vi "Performance Test.vi"() -> ()   [LabVIEW 2021]
uses:
  CIFChannels/Typedef/Direction.ctl
  CIF_NIChn_Fifo_Power.lvclass
  D:/dev/CIF-LVCore/src/Channels/CIFChannels/CIFChannels.lvclass
  D:/dev/CIF-LVCore/src/Channels/CIF_NIChn/NIChn/CIF_NIChn.lvclass
  ChannelCommon/typedef/FIFO Config.ctl
  <vilib>/Platform/TimedLoop/XDataNode/timing_clust.ctl
  <vilib>/Platform/TimedLoop/XDataNode/nitl_modes.ctl
  <vilib>/Platform/TimedLoop/XDataNode/wakeup.ctl
  ChannelCommon/typedef/Datatype Waveform.ctl
  CIF_NIChn_Fifo_Power.lvclass/CIF_NIChn_Fifo_Power.ctl
  ChannelCommon/CIFFIFO/CIFfifo.lvclass/CIFfifo.ctl
  NIChn/CIF_NIChn.lvclass/CIF_NIChn.ctl
  CIFChannels/CIFChannels.lvclass/CIFChannels.ctl
  CIFCore/Common/Utilities/Add Error.vi
  SubVIs/Add Error.vi
  <vilib>/CIFChannels/Top Level/Write Variable Length U8 Array.vi
  NIChn/Accessors/Read CIF Channel.vi
  NIChn/Accessors/Write CIF Channel.vi
  SubVIs/Flatten.vi
  ChannelCommon/CIFFIFO/Accessors/Read Length.vi
  NIChn/SubVIs/Check Disconnect.vi
  <vilib>/CIFChannels/Top Level/Read Variable Length U8 Array.vi
  SubVIs/Unflatten.vi
  CIFChannels/Accessors/Read Channel State.vi
  CIFChannels/Accessors/Read Direction.vi
  CIFCore/Common/Utilities/Append Error Location.vi
  <vilib>/CIFChannels/SubVIs/Get dll Path.vi
  ChannelCommon/CIFFIFO/Utilities/Update Header.vi
  ChannelCommon/CIFFIFO/Flatten/Waveform Flatten.vi
  ChannelCommon/CIFFIFO/Accessors/Write T0.vi
  ChannelCommon/CIFFIFO/Accessors/Write T_Out.vi
  CIFChannels/Accessors/Write Channel State.vi
  CIFChannels/Accessors/Read Disconnect Behavior.vi
  <vilib>/CIFChannels/Top Level/Read Variable Length U8 Array.vi/81056090-23cf-424a-a716-29db01c8ef1b.vi
  <vilib>/CIFChannels/Top Level/Read Variable Length U8 Array.vi/6610cd62-0a6d-4591-8fd4-6453482a4bc1.vi
  <vilib>/CIFChannels/Top Level/Read Variable Length U8 Array.vi/93d598b0-524b-4f76-9570-a74a86ef2c6f.vi
  ChannelCommon/CIFFIFO/Accessors/Write Timeout.vi
  ChannelCommon/CIFFIFO/Flatten/Waveform Unflatten.vi
  ChannelCommon/CIFFIFO/Accessors/Read Header.vi
  ChannelCommon/CIFFIFO/Accessors/Write Header.vi
  ChannelCommon/Utilities/Flatten Header.vi
  ChannelCommon/CIFFIFO/Flatten/Waveform Flatten.vi/6fdbece9-bad6-4a8e-9bf7-fe1528478dd6.vi
  ChannelCommon/CIFFIFO/Flatten/Waveform Flatten.vi/d5e54e4f-7f1a-40ef-960c-6b2cd585230c.vi
  ChannelCommon/CIFFIFO/Flatten/Waveform Flatten.vi/a071385d-aa0c-48d2-a5ce-3b08816305e6.vi
  ChannelCommon/CIFFIFO/Accessors/Write Payload Length.vi
  <vilib>/CIFChannels/Top Level/Read Variable Length U8 Array.vi/81056090-23cf-424a-a716-29db01c8ef1b.vi/4bc1c15b-36ab-481f-b8dd-c64075ce723a.vi
  <vilib>/CIFChannels/Top Level/Read Variable Length U8 Array.vi/81056090-23cf-424a-a716-29db01c8ef1b.vi/d83cb72b-7713-41fc-a3d1-682de79cf574.vi
  <vilib>/CIFChannels/Top Level/Read Variable Length U8 Array.vi/6610cd62-0a6d-4591-8fd4-6453482a4bc1.vi/c28b0ead-42ad-4072-80a2-aca7f2bd7ce3.vi
  <vilib>/CIFChannels/Top Level/Read Variable Length U8 Array.vi/93d598b0-524b-4f76-9570-a74a86ef2c6f.vi/4bc1c15b-36ab-481f-b8dd-c64075ce723a.vi
  <vilib>/CIFChannels/Top Level/Read Variable Length U8 Array.vi/93d598b0-524b-4f76-9570-a74a86ef2c6f.vi/d83cb72b-7713-41fc-a3d1-682de79cf574.vi
  ChannelCommon/Utilities/Unflatten Header.vi
  ChannelCommon/CIFFIFO/Flatten/Waveform Flatten.vi/6fdbece9-bad6-4a8e-9bf7-fe1528478dd6.vi/c28b0ead-42ad-4072-80a2-aca7f2bd7ce3.vi
  ChannelCommon/CIFFIFO/Flatten/Waveform Flatten.vi/d5e54e4f-7f1a-40ef-960c-6b2cd585230c.vi/c28b0ead-42ad-4072-80a2-aca7f2bd7ce3.vi
  ChannelCommon/CIFFIFO/Flatten/Waveform Flatten.vi/a071385d-aa0c-48d2-a5ce-3b08816305e6.vi/c28b0ead-42ad-4072-80a2-aca7f2bd7ce3.vi
  NIChn/CIF_NIChn.lvclass
  ChannelCommon/Utilities/Update Time.vi
  <vilib>/Platform/TimedLoop/XDataNode/XDataNode.xnode
  <vilib>/Platform/TimedLoop/XDataNode/XDNodeRunTimeDep.lvlib
  CIFChannels/CIFChannels.lvclass
  ChannelCommon/ChannelCommon.lvlib
panel:
  out "avg big channel":dbl
  out "max big channel":dbl
  out "timed out? 4":bool
  out "avg TO":dbl
  out "max TO":dbl
  out "timed out? 3":bool
  out "avg Direct":dbl
  out "max Direct":dbl
  out "timed out? 2":bool
  out "timed out?":bool
  out "avg channel":dbl
  out "max channel":dbl
  out "pass":bool
  out "error out":errorcluster
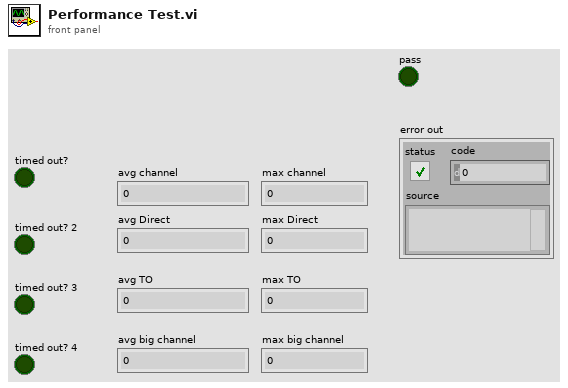
[diagram p1: front panel]
types:
  T1 = typedef "ChannelCommon.lvlib/FIFO Config.ctl" = cluster{"Depth":u64, "Flags":u64, "ClockID":u8}
  T2 = typedef "CIFChannels.lvclass/Direction.ctl" = enum16{"Publisher", "Subscriber"}
  T3 = typedef "ChannelCommon.lvlib/Datatype Waveform.ctl" = cluster{"measurement":dbl[], "dT":dbl, "Timestamp":u64}
  T4 = typedef "XDNodeRunTimeDep.lvlib/timing_clust.ctl" = cluster{"Expected End [f-1]":u64, "Actual End [f-1]":u64, "Finished Late? [f-1]":bool, "Expected End [i-1]":u64, "Actual End [i-1]":u64, "Finished Late? [i-1]":bool, "Expected Start [i]":u64, "Actual Start [i]":u64, "Expected Start [f]":u64, "Actual Start [f]":u64, "Source Name":string, "Structure Name":string, "Period":i64, "Deadline":i64, "Offset":i64, "Start":i64, "Priority":i32, "Timeout":i32, "Mode":T5, "Wakeup Reason":T6, "Error":errorcluster, "Source Type":string, "Secondary Source Type":string, "Global End Time":u64, "Global Start Time":u64, "Frame Duration":u64, "Iteration Duration":u64, "Assigned CPU":i32, "I/O Scan Engine Mode":u32}
  T5 = typedef "XDNodeRunTimeDep.lvlib/nitl_modes.ctl" = enum32{"No Change", "Process missed periods, maintain original phase", "Discard missed periods, maintain original phase", "Process missed periods, ignore original phase", "Discard missed periods, ignore original phase"}
  T6 = typedef "XDNodeRunTimeDep.lvlib/wakeup.ctl" = enum32{"Normal", "Aborted", "Asynchronous wakeup", "Timing source error", "Timed loop error", "Timeout"}
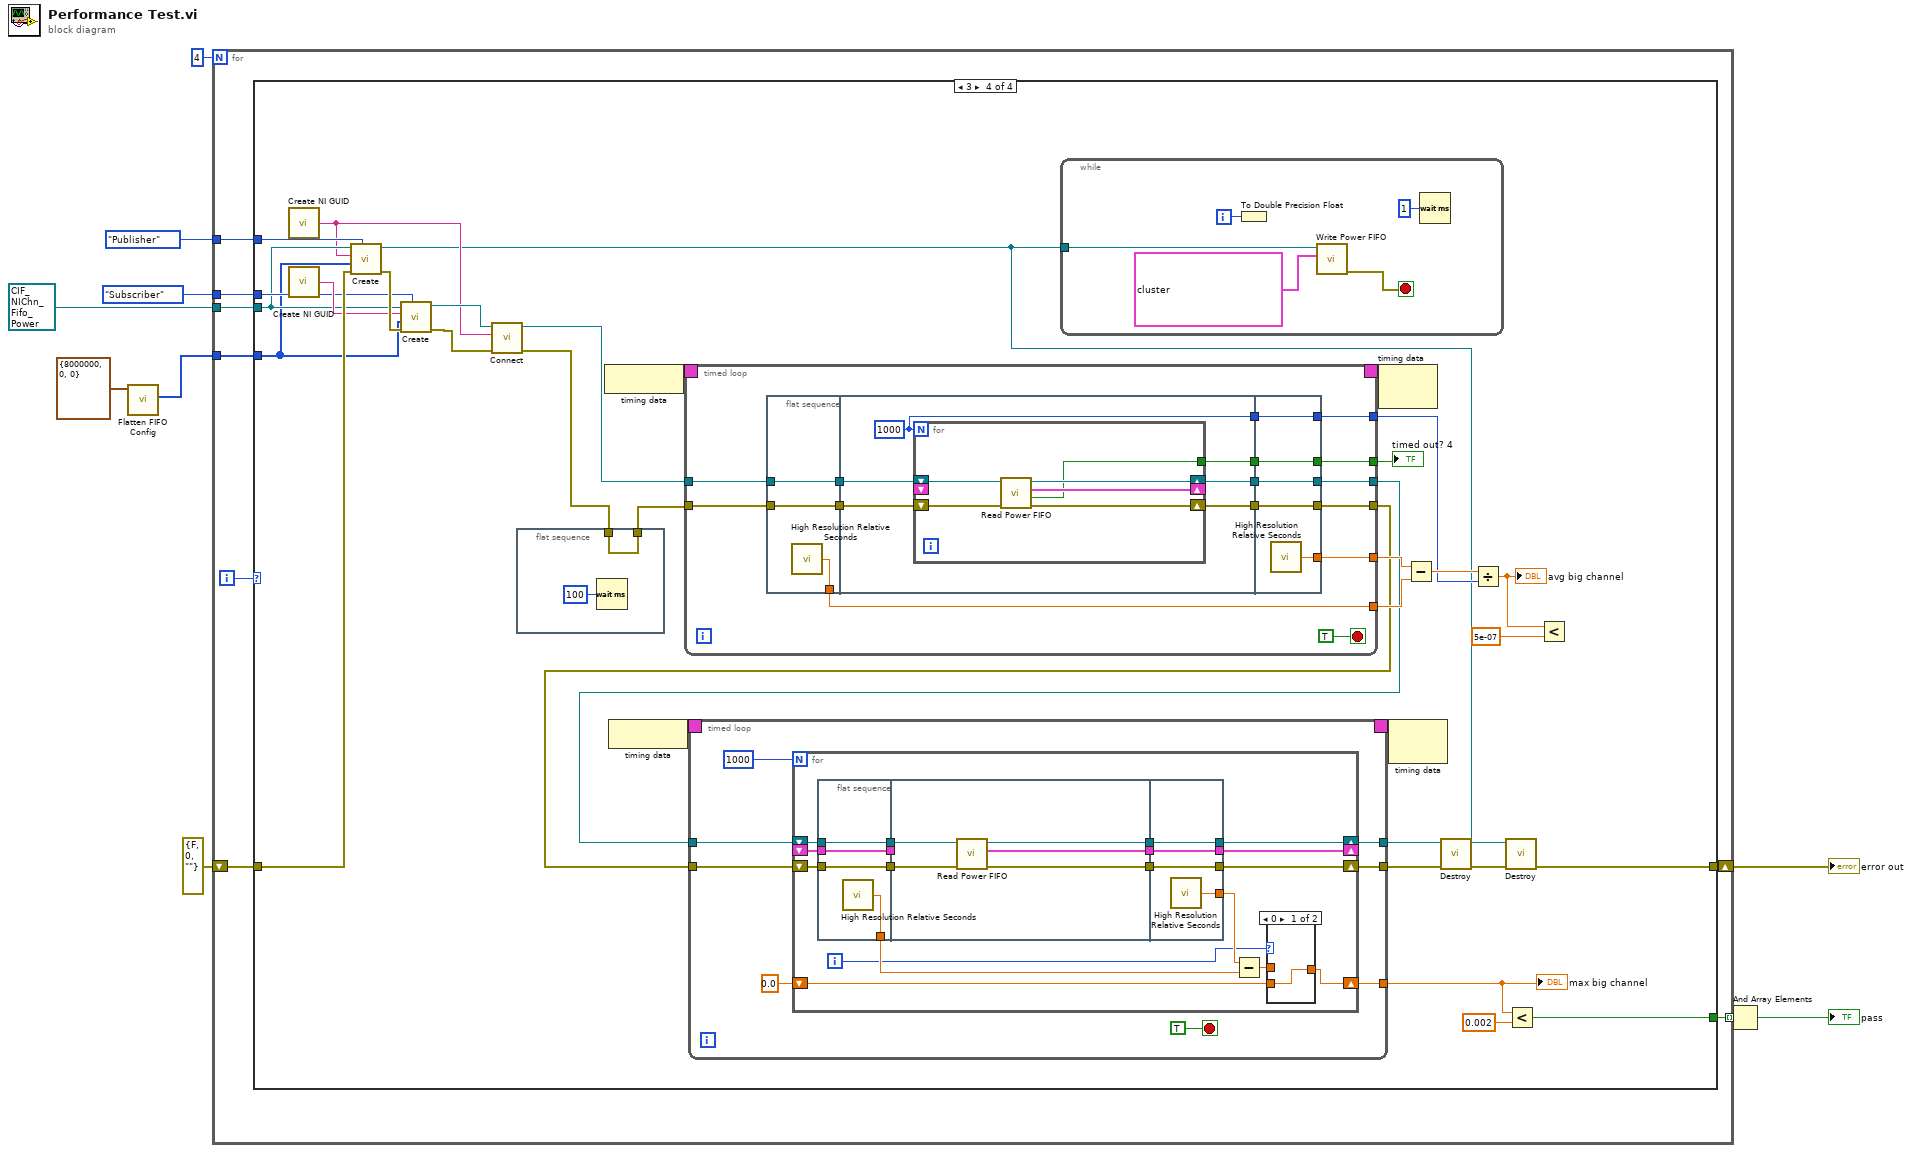
[diagram p0: block diagram]
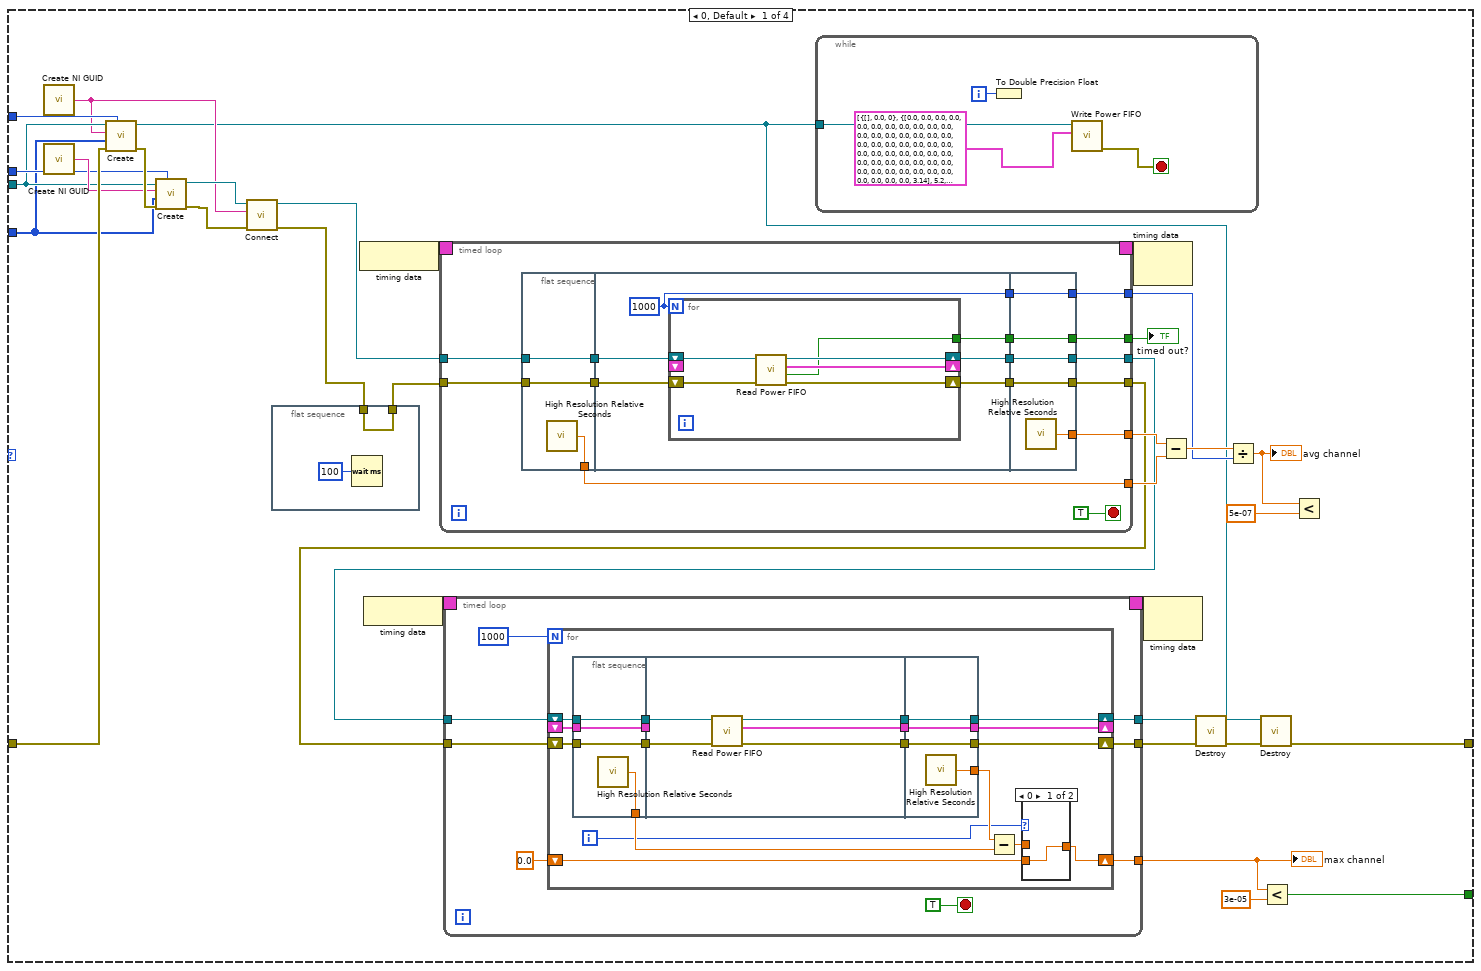
[diagram p2: hidden frame]
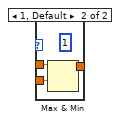
[diagram p3: hidden frame]
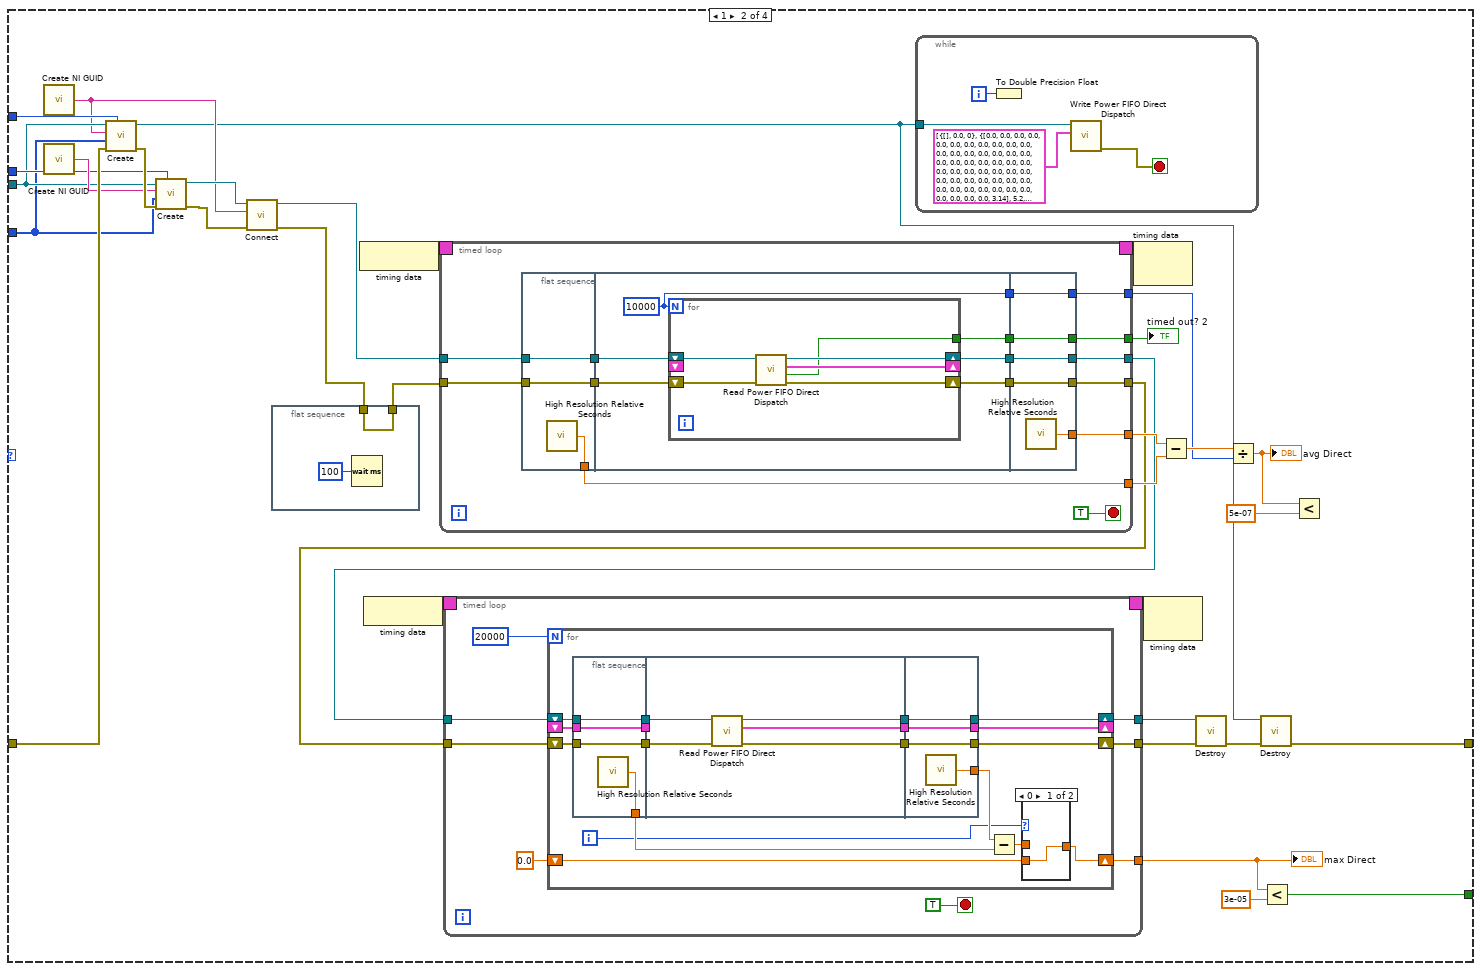
[diagram p4: hidden frame]
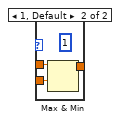
[diagram p5: hidden frame]
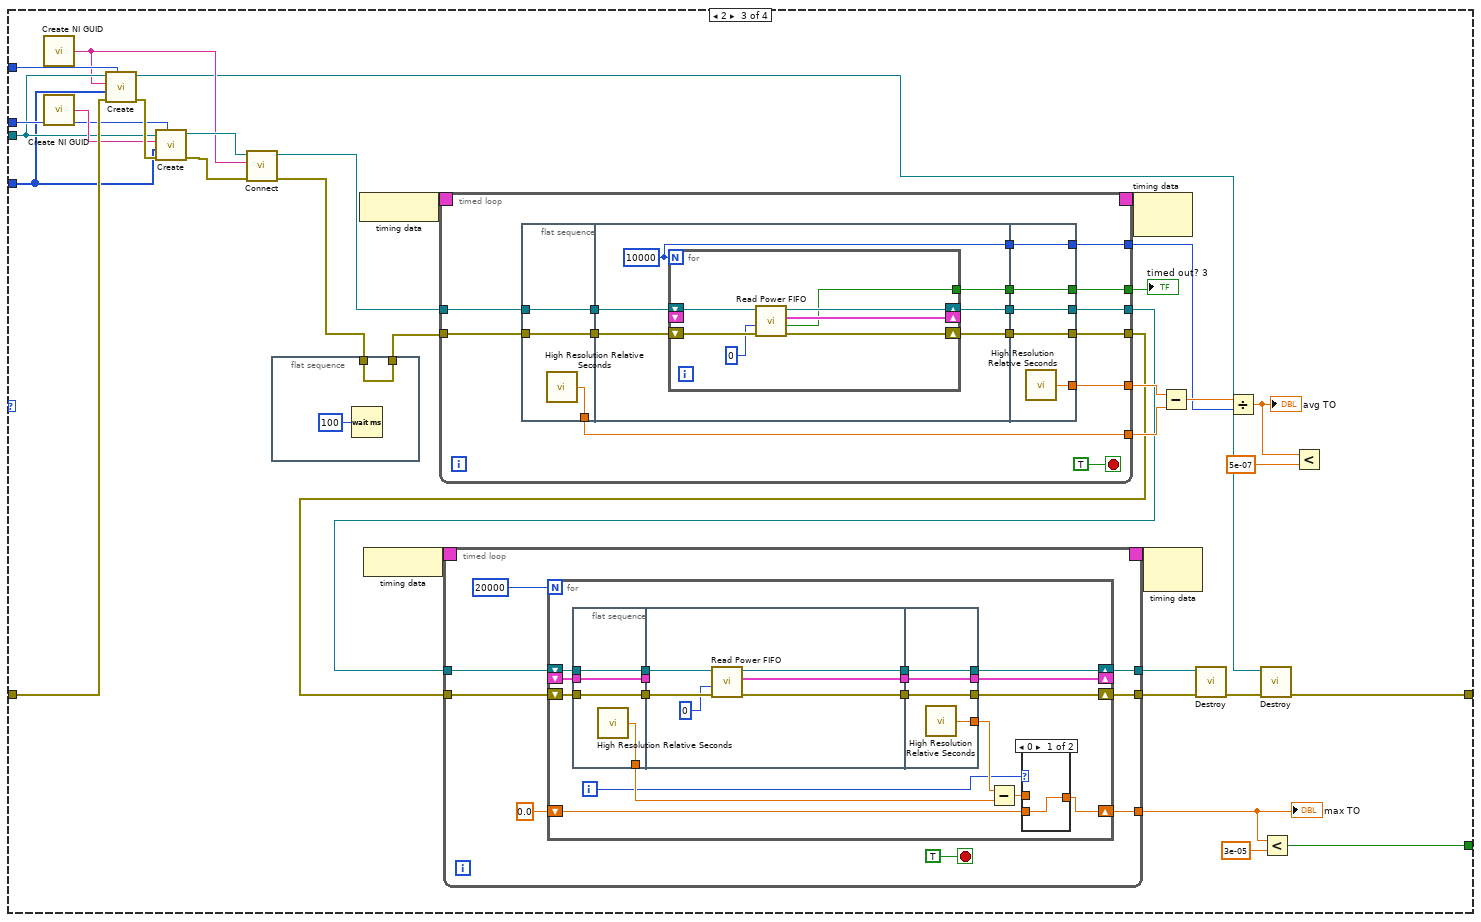
[diagram p6: hidden frame]
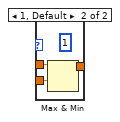
[diagram p7: hidden frame]
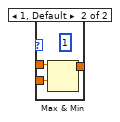
[diagram p8: hidden frame]
diagram:
  n1 = call "Flatten FIFO Config.vi"("FIFO Config in"=T1 {"Depth"=8000000, "Flags"=0, "ClockID"=0}) -> ("Flattened Data out"=w2:u8[])  [unwired: 8 in, 2 out]
  n2 = for {
    N: 4 -> [_]
    tunnel: [w18] -> w8 mode=indexing
    shift-right: [w17] -> w10
    shift-left: errorcluster {"status"=FALSE, "code"=0, "source"=""} ("error out") -> [w15]
    tunnel: Direction."Publisher" ("Direction") -> [w14]
    tunnel: Direction."Subscriber" ("Direction") -> [w13]
    tunnel: refnum<class "CIF_NIChn_Fifo_Power.lvclass"> refnum ("CIF_NIChn_Fifo_Power.lvclass") -> [w12]
    tunnel: w2 -> [w11]
    i -> [w16]
    n3 = case shown="3" w16 {
      tunnel: [w38 w164 w290 w414] -> w18
      tunnel: [w22 w148 w274 w398] -> w17
      tunnel: w15 -> [w36 w162 w288 w412]
      tunnel: w14 -> [w34 w160 w286 w410]
      tunnel: w13 -> [w33 w159 w285 w409]
      tunnel: w12 -> [w32 w158 w284 w408]
      tunnel: w11 -> [w28 w154 w280 w404]
      frame 0, Default {
        n4 = call <vilib>:"Create NI GUID.vi"() -> ("NI GUID"=w30:string)
        n5 = call <vilib>:"Create NI GUID.vi"() -> ("NI GUID"=w35:string)
        n6 = call-dynamic "Create.vi"("Direction"=w34, "error in (no error)"=w36, "Custom Config Data"=w28, "Name"=w30, "CIFTag in"=w32) -> ("error out"=w37:errorcluster, "CIFTag out"=w23:refnum<class "CIF_NIChn_Fifo_Power.lvclass">)  [unwired: 5 in]
        n7 = call-dynamic "Create.vi"("Direction"=w33, "error in (no error)"=w37, "Custom Config Data"=w28, "Name"=w35, "CIFTag in"=w32) -> ("error out"=w29:errorcluster, "CIFTag out"=w31:refnum<class "CIF_NIChn_Fifo_Power.lvclass">)  [unwired: 5 in]
        n8 = call-dynamic "Connect.vi"("error in (no error)"=w29, "Connection Name"=w30, "CIFTag in"=w31) -> ("error out"=w21:errorcluster, "CIFTag out"=w27:refnum<class "CIF_NIChn_Fifo_Power.lvclass">)  [unwired: 7 in]
        n9 = flat-sequence {
          tunnel: w21 -> [w54]
          tunnel: [w54] -> w20
          frame #0 {
            n10 = Wait (ms)(milliseconds to wait=u32 100) -> ()  [unwired: 1 out]
          }
        }
        n11 = node-c288() -> (w52:T4)
        n12 = node-c288() -> (w50:T4)
        n13 = timed-loop {
          timing: w52 -> [_]
          timing-out: [_] -> w51
          tunnel: w27 -> [w120]
          tunnel: w20 -> [w119]
          tunnel: [w115] -> w44
          tunnel: [w113] -> w43
          tunnel: [w111] -> w48
          tunnel: [w110] -> w47
          tunnel: [w109] -> w45
          tunnel: [w107] -> w19
          stop <- TRUE stop-if-true
          n14 = flat-sequence {
            tunnel: w119 -> [w122]
            tunnel: w120 -> [w123]
            tunnel: [w123] -> w117
            tunnel: [w122] -> w116
            tunnel: [w121] -> w110
            tunnel: w117 -> [w129]
            tunnel: w116 -> [w128]
            tunnel: [w127] -> w114
            tunnel: [w126] -> w112
            tunnel: [w125] -> w108
            tunnel: [w124] -> w106
            tunnel: [w140] -> w115
            tunnel: w114 -> [w140]
            tunnel: [w139] -> w113
            tunnel: w112 -> [w139]
            tunnel: [w138] -> w111
            tunnel: [w137] -> w109
            tunnel: w108 -> [w137]
            tunnel: [w136] -> w107
            tunnel: w106 -> [w136]
            frame #0 {
              n15 = call <vilib>:"High Resolution Relative Seconds.vi"() -> ("relative seconds"=w121:dbl)
            }
            frame #1 {
              w125 = 1000
              n16 = for {
                N: w125 -> [_]
                shift-right: [w134] -> w127
                shift-left: w129 -> [w135]
                shift-right: [w132] -> w126
                shift-left: w128 -> [w133]
                shift-right: [w131] -> _
                shift-left: _ -> [_]
                tunnel: [w130] -> w124
                n17 = call-dynamic "Read Power FIFO.vi"("error in (no error)"=w133, "CIFTag in"=w135) -> ("error out"=w132:errorcluster, "timed out?"=w130:bool, "Data out"=w131:T3[], "CIFTag out"=w134:refnum<class "CIF_NIChn_Fifo_Power.lvclass">)  [unwired: 5 in, 1 out]
              }
            }
            frame #2 {
              n18 = call <vilib>:"High Resolution Relative Seconds.vi"() -> ("relative seconds"=w138:dbl)
            }
          }
        }
        "timed out?" <- w19
        n19 = timed-loop {
          timing: w50 -> [_]
          timing-out: [_] -> w49
          tunnel: w44 -> [w66]
          tunnel: w43 -> [w65]
          tunnel: [w63] -> w26
          tunnel: [w62] -> w25
          tunnel: [w59] -> w40
          stop <- TRUE stop-if-true
          n20 = for {
            N: 1000 -> [_]
            shift-right: [w78] -> w63
            shift-left: w66 -> [w80]
            shift-right: [w77] -> w62
            shift-left: w65 -> [w79]
            shift-right: [w71] -> w59
            shift-left: 0.0 -> [w72]
            shift-right: [w70] -> _
            shift-left: _ -> [w76]
            i -> [w68]
            n21 = flat-sequence {
              tunnel: w79 -> [w91]
              tunnel: w80 -> [w92]
              tunnel: [w92] -> w84
              tunnel: [w91] -> w83
              tunnel: [w90] -> w74
              tunnel: w76 -> [w89]
              tunnel: [w89] -> w82
              tunnel: w84 -> [w97]
              tunnel: w83 -> [w95]
              tunnel: [w96] -> w81
              tunnel: w82 -> [_]
              tunnel: [w93] -> w69
              tunnel: [w94] -> w67
              tunnel: [w101] -> w78
              tunnel: w81 -> [w101]
              tunnel: [w100] -> w77
              tunnel: [w99] -> w75
              tunnel: [w98] -> w70
              tunnel: w69 -> [w98]
              tunnel: w67 -> [w100]
              frame #0 {
                n22 = call <vilib>:"High Resolution Relative Seconds.vi"() -> ("relative seconds"=w90:dbl)
              }
              frame #1 {
                n23 = call-dynamic "Read Power FIFO.vi"("error in (no error)"=w95, "CIFTag in"=w97) -> ("error out"=w94:errorcluster, "Data out"=w93:T3[], "CIFTag out"=w96:refnum<class "CIF_NIChn_Fifo_Power.lvclass">)  [unwired: 5 in, 2 out]
              }
              frame #2 {
                n24 = call <vilib>:"High Resolution Relative Seconds.vi"() -> ("relative seconds"=w99:dbl)
              }
            }
            n25 = Subtract(x=w75, y=w74) -> (x-y=w73:dbl)
            n26 = case shown="0" w68 {
              tunnel: w73 -> [_ w88]
              tunnel: w72 -> [w85 w87]
              tunnel: [w85 w86] -> w71
              frame 0 {
              }
              frame 1, Default {
                (unwired) u32 1 ("milliseconds to wait")
                n27 = Max & Min(x=w88, y=w87) -> (max(x,y)=w86:dbl)  [unwired: 1 out]
              }
            }
          }
        }
        "max channel" <- w40
        n28 = while {
          tunnel: w23 -> [w57]
          i -> [w58]
          stop <- w56 stop-if-true
          n29 = To Double Precision Float(number=w58) -> ()  [unwired: 1 out]
          n30 = call-dynamic "Write Power FIFO.vi"("Data In"=T3[] [{"measurement"=[], "dT"=0.0, "Timestamp"=0}, {"measurement"=[0.0, 0.0, 0.0, 0.0, 0.0, 0.0, 0.0, 0.0, 0.0, 0.0, 0.0, 0.0, 0.0, 0.0, 0.0, 0.0, 0.0, 0.0, 0.0, 0.0, 0.0, 0.0, 0.0, 0.0, 0.0, 0.0, 0.0, 0.0, 0.0, 0.0, 0.0, 0.0, 0.0, 0.0, 0.0, 0.0, 0.0, 0.0, 0.0, 0.0, 0.0, 0.0, 0.0, 0.0, 0.0, 0.0, 0.0, 0.0, 0.0, 0.0, 3.14], "dT"=5.2, "Timestamp"=523}], "CIFTag in"=w57) -> ("error out"=w56:errorcluster)  [unwired: 6 in, 3 out]
        }
        n31 = node-c288(w51) -> ()  [unwired: 1 out]
        n32 = node-c288(w49) -> ()  [unwired: 1 out]
        n33 = Subtract(x=w48, y=w47) -> (x-y=w46:dbl)
        n34 = call-dynamic "Destroy.vi"("error in (no error)"=w25, "CIFTag in"=w26) -> ("error out"=w24:errorcluster)  [unwired: 8 in, 1 out]
        n35 = Divide(x=w46, y=w45) -> (x/y=w42:dbl)
        "avg channel" <- w42
        n36 = call-dynamic "Destroy.vi"("error in (no error)"=w24, "CIFTag in"=w23) -> ("error out"=w22:errorcluster)  [unwired: 8 in, 1 out]
        n37 = Less?(x=w40, y=3e-05) -> (x < y?=w38:bool)
        n38 = Less?(x=w42, y=5e-07) -> ()  [unwired: 1 out]
      }
      frame 1 {
        n39 = call <vilib>:"Create NI GUID.vi"() -> ("NI GUID"=w156:string)
        n40 = call <vilib>:"Create NI GUID.vi"() -> ("NI GUID"=w161:string)
        n41 = call-dynamic "Create.vi"("Direction"=w160, "error in (no error)"=w162, "Custom Config Data"=w154, "Name"=w156, "CIFTag in"=w158) -> ("error out"=w163:errorcluster, "CIFTag out"=w149:refnum<class "CIF_NIChn_Fifo_Power.lvclass">)  [unwired: 5 in]
        n42 = call-dynamic "Create.vi"("Direction"=w159, "error in (no error)"=w163, "Custom Config Data"=w154, "Name"=w161, "CIFTag in"=w158) -> ("error out"=w155:errorcluster, "CIFTag out"=w157:refnum<class "CIF_NIChn_Fifo_Power.lvclass">)  [unwired: 5 in]
        n43 = call-dynamic "Connect.vi"("error in (no error)"=w155, "Connection Name"=w156, "CIFTag in"=w157) -> ("error out"=w147:errorcluster, "CIFTag out"=w153:refnum<class "CIF_NIChn_Fifo_Power.lvclass">)  [unwired: 7 in]
        n44 = flat-sequence {
          tunnel: w147 -> [w180]
          tunnel: [w180] -> w146
          frame #0 {
            n45 = Wait (ms)(milliseconds to wait=u32 100) -> ()  [unwired: 1 out]
          }
        }
        n46 = node-c288() -> (w178:T4)
        n47 = node-c288() -> (w176:T4)
        n48 = timed-loop {
          timing: w178 -> [_]
          timing-out: [_] -> w177
          tunnel: w153 -> [w246]
          tunnel: w146 -> [w245]
          tunnel: [w241] -> w170
          tunnel: [w239] -> w169
          tunnel: [w237] -> w174
          tunnel: [w236] -> w173
          tunnel: [w235] -> w171
          tunnel: [w233] -> w145
          stop <- TRUE stop-if-true
          n49 = flat-sequence {
            tunnel: w245 -> [w248]
            tunnel: w246 -> [w249]
            tunnel: [w249] -> w243
            tunnel: [w248] -> w242
            tunnel: [w247] -> w236
            tunnel: w243 -> [w255]
            tunnel: w242 -> [w254]
            tunnel: [w253] -> w240
            tunnel: [w252] -> w238
            tunnel: [w251] -> w234
            tunnel: [w250] -> w232
            tunnel: [w266] -> w241
            tunnel: w240 -> [w266]
            tunnel: [w265] -> w239
            tunnel: w238 -> [w265]
            tunnel: [w264] -> w237
            tunnel: [w263] -> w235
            tunnel: w234 -> [w263]
            tunnel: [w262] -> w233
            tunnel: w232 -> [w262]
            frame #0 {
              n50 = call <vilib>:"High Resolution Relative Seconds.vi"() -> ("relative seconds"=w247:dbl)
            }
            frame #1 {
              w251 = 10000
              n51 = for {
                N: w251 -> [_]
                shift-right: [w260] -> w253
                shift-left: w255 -> [w261]
                shift-right: [w258] -> w252
                shift-left: w254 -> [w259]
                shift-right: [w257] -> _
                shift-left: _ -> [_]
                tunnel: [w256] -> w250
                n52 = call "Read Power FIFO Direct Dispatch.vi"("error in (no error)"=w259, "CIFTag in"=w261) -> ("error out"=w258:errorcluster, "timed out?"=w256:bool, "Data out"=w257:T3[], "CIFTag out"=w260:refnum<class "CIF_NIChn_Fifo_Power.lvclass">)  [unwired: 5 in, 1 out]
              }
            }
            frame #2 {
              n53 = call <vilib>:"High Resolution Relative Seconds.vi"() -> ("relative seconds"=w264:dbl)
            }
          }
        }
        "timed out? 2" <- w145
        n54 = timed-loop {
          timing: w176 -> [_]
          timing-out: [_] -> w175
          tunnel: w170 -> [w192]
          tunnel: w169 -> [w191]
          tunnel: [w189] -> w152
          tunnel: [w188] -> w151
          tunnel: [w185] -> w166
          stop <- TRUE stop-if-true
          n55 = for {
            N: 20000 -> [_]
            shift-right: [w204] -> w189
            shift-left: w192 -> [w206]
            shift-right: [w203] -> w188
            shift-left: w191 -> [w205]
            shift-right: [w197] -> w185
            shift-left: 0.0 -> [w198]
            shift-right: [w196] -> _
            shift-left: _ -> [w202]
            i -> [w194]
            n56 = flat-sequence {
              tunnel: w205 -> [w217]
              tunnel: w206 -> [w218]
              tunnel: [w218] -> w210
              tunnel: [w217] -> w209
              tunnel: [w216] -> w200
              tunnel: w202 -> [w215]
              tunnel: [w215] -> w208
              tunnel: w210 -> [w223]
              tunnel: w209 -> [w221]
              tunnel: [w222] -> w207
              tunnel: w208 -> [_]
              tunnel: [w219] -> w195
              tunnel: [w220] -> w193
              tunnel: [w227] -> w204
              tunnel: w207 -> [w227]
              tunnel: [w226] -> w203
              tunnel: [w225] -> w201
              tunnel: [w224] -> w196
              tunnel: w195 -> [w224]
              tunnel: w193 -> [w226]
              frame #0 {
                n57 = call <vilib>:"High Resolution Relative Seconds.vi"() -> ("relative seconds"=w216:dbl)
              }
              frame #1 {
                n58 = call "Read Power FIFO Direct Dispatch.vi"("error in (no error)"=w221, "CIFTag in"=w223) -> ("error out"=w220:errorcluster, "Data out"=w219:T3[], "CIFTag out"=w222:refnum<class "CIF_NIChn_Fifo_Power.lvclass">)  [unwired: 5 in, 2 out]
              }
              frame #2 {
                n59 = call <vilib>:"High Resolution Relative Seconds.vi"() -> ("relative seconds"=w225:dbl)
              }
            }
            n60 = Subtract(x=w201, y=w200) -> (x-y=w199:dbl)
            n61 = case shown="0" w194 {
              tunnel: w199 -> [_ w214]
              tunnel: w198 -> [w211 w213]
              tunnel: [w211 w212] -> w197
              frame 0 {
              }
              frame 1, Default {
                (unwired) u32 1 ("milliseconds to wait")
                n62 = Max & Min(x=w214, y=w213) -> (max(x,y)=w212:dbl)  [unwired: 1 out]
              }
            }
          }
        }
        "max Direct" <- w166
        n63 = while {
          tunnel: w149 -> [w183]
          i -> [w184]
          stop <- w182 stop-if-true
          n64 = To Double Precision Float(number=w184) -> ()  [unwired: 1 out]
          n65 = call "Write Power FIFO Direct Dispatch.vi"("Data In"=T3[] [{"measurement"=[], "dT"=0.0, "Timestamp"=0}, {"measurement"=[0.0, 0.0, 0.0, 0.0, 0.0, 0.0, 0.0, 0.0, 0.0, 0.0, 0.0, 0.0, 0.0, 0.0, 0.0, 0.0, 0.0, 0.0, 0.0, 0.0, 0.0, 0.0, 0.0, 0.0, 0.0, 0.0, 0.0, 0.0, 0.0, 0.0, 0.0, 0.0, 0.0, 0.0, 0.0, 0.0, 0.0, 0.0, 0.0, 0.0, 0.0, 0.0, 0.0, 0.0, 0.0, 0.0, 0.0, 0.0, 0.0, 0.0, 3.14], "dT"=5.2, "Timestamp"=523}], "CIFTag in"=w183) -> ("error out"=w182:errorcluster)  [unwired: 6 in, 3 out]
        }
        n66 = node-c288(w177) -> ()  [unwired: 1 out]
        n67 = node-c288(w175) -> ()  [unwired: 1 out]
        n68 = Subtract(x=w174, y=w173) -> (x-y=w172:dbl)
        n69 = call-dynamic "Destroy.vi"("error in (no error)"=w151, "CIFTag in"=w152) -> ("error out"=w150:errorcluster)  [unwired: 8 in, 1 out]
        n70 = Divide(x=w172, y=w171) -> (x/y=w168:dbl)
        "avg Direct" <- w168
        n71 = call-dynamic "Destroy.vi"("error in (no error)"=w150, "CIFTag in"=w149) -> ("error out"=w148:errorcluster)  [unwired: 8 in, 1 out]
        n72 = Less?(x=w166, y=3e-05) -> (x < y?=w164:bool)
        n73 = Less?(x=w168, y=5e-07) -> ()  [unwired: 1 out]
      }
      frame 2 {
        n74 = call <vilib>:"Create NI GUID.vi"() -> ("NI GUID"=w282:string)
        n75 = call <vilib>:"Create NI GUID.vi"() -> ("NI GUID"=w287:string)
        n76 = call-dynamic "Create.vi"("Direction"=w286, "error in (no error)"=w288, "Custom Config Data"=w280, "Name"=w282, "CIFTag in"=w284) -> ("error out"=w289:errorcluster, "CIFTag out"=w275:refnum<class "CIF_NIChn_Fifo_Power.lvclass">)  [unwired: 5 in]
        n77 = call-dynamic "Create.vi"("Direction"=w285, "error in (no error)"=w289, "Custom Config Data"=w280, "Name"=w287, "CIFTag in"=w284) -> ("error out"=w281:errorcluster, "CIFTag out"=w283:refnum<class "CIF_NIChn_Fifo_Power.lvclass">)  [unwired: 5 in]
        n78 = call-dynamic "Connect.vi"("error in (no error)"=w281, "Connection Name"=w282, "CIFTag in"=w283) -> ("error out"=w273:errorcluster, "CIFTag out"=w279:refnum<class "CIF_NIChn_Fifo_Power.lvclass">)  [unwired: 7 in]
        n79 = flat-sequence {
          tunnel: w273 -> [w306]
          tunnel: [w306] -> w272
          frame #0 {
            n80 = Wait (ms)(milliseconds to wait=u32 100) -> ()  [unwired: 1 out]
          }
        }
        n81 = node-c288() -> (w304:T4)
        n82 = node-c288() -> (w302:T4)
        n83 = timed-loop {
          timing: w304 -> [_]
          timing-out: [_] -> w303
          tunnel: w279 -> [w369]
          tunnel: w272 -> [w368]
          tunnel: [w364] -> w296
          tunnel: [w362] -> w295
          tunnel: [w360] -> w300
          tunnel: [w359] -> w299
          tunnel: [w358] -> w297
          tunnel: [w356] -> w271
          stop <- TRUE stop-if-true
          n84 = flat-sequence {
            tunnel: w368 -> [w371]
            tunnel: w369 -> [w372]
            tunnel: [w372] -> w366
            tunnel: [w371] -> w365
            tunnel: [w370] -> w359
            tunnel: w366 -> [w378]
            tunnel: w365 -> [w377]
            tunnel: [w376] -> w363
            tunnel: [w375] -> w361
            tunnel: [w374] -> w357
            tunnel: [w373] -> w355
            tunnel: [w390] -> w364
            tunnel: w363 -> [w390]
            tunnel: [w389] -> w362
            tunnel: w361 -> [w389]
            tunnel: [w388] -> w360
            tunnel: [w387] -> w358
            tunnel: w357 -> [w387]
            tunnel: [w386] -> w356
            tunnel: w355 -> [w386]
            frame #0 {
              n85 = call <vilib>:"High Resolution Relative Seconds.vi"() -> ("relative seconds"=w370:dbl)
            }
            frame #1 {
              w374 = 10000
              n86 = for {
                N: w374 -> [_]
                shift-right: [w384] -> w376
                shift-left: w378 -> [w385]
                shift-right: [w382] -> w375
                shift-left: w377 -> [w383]
                shift-right: [w381] -> _
                shift-left: _ -> [_]
                tunnel: [w380] -> w373
                n87 = call-dynamic "Read Power FIFO.vi"("error in (no error)"=w383, "Timeout (ms)"=0, "CIFTag in"=w385) -> ("error out"=w382:errorcluster, "timed out?"=w380:bool, "Data out"=w381:T3[], "CIFTag out"=w384:refnum<class "CIF_NIChn_Fifo_Power.lvclass">)  [unwired: 4 in, 1 out]
              }
            }
            frame #2 {
              n88 = call <vilib>:"High Resolution Relative Seconds.vi"() -> ("relative seconds"=w388:dbl)
            }
          }
        }
        "timed out? 3" <- w271
        n89 = timed-loop {
          timing: w302 -> [_]
          timing-out: [_] -> w301
          tunnel: w296 -> [w314]
          tunnel: w295 -> [w313]
          tunnel: [w311] -> w278
          tunnel: [w310] -> w277
          tunnel: [w307] -> w292
          stop <- TRUE stop-if-true
          n90 = for {
            N: 20000 -> [_]
            shift-right: [w326] -> w311
            shift-left: w314 -> [w328]
            shift-right: [w325] -> w310
            shift-left: w313 -> [w327]
            shift-right: [w319] -> w307
            shift-left: 0.0 -> [w320]
            shift-right: [w318] -> _
            shift-left: _ -> [w324]
            i -> [w316]
            n91 = flat-sequence {
              tunnel: w327 -> [w339]
              tunnel: w328 -> [w340]
              tunnel: [w340] -> w332
              tunnel: [w339] -> w331
              tunnel: [w338] -> w322
              tunnel: w324 -> [w337]
              tunnel: [w337] -> w330
              tunnel: w332 -> [w346]
              tunnel: w331 -> [w344]
              tunnel: [w345] -> w329
              tunnel: w330 -> [_]
              tunnel: [w342] -> w317
              tunnel: [w343] -> w315
              tunnel: [w350] -> w326
              tunnel: w329 -> [w350]
              tunnel: [w349] -> w325
              tunnel: [w348] -> w323
              tunnel: [w347] -> w318
              tunnel: w317 -> [w347]
              tunnel: w315 -> [w349]
              frame #0 {
                n92 = call <vilib>:"High Resolution Relative Seconds.vi"() -> ("relative seconds"=w338:dbl)
              }
              frame #1 {
                n93 = call-dynamic "Read Power FIFO.vi"("error in (no error)"=w344, "Timeout (ms)"=0, "CIFTag in"=w346) -> ("error out"=w343:errorcluster, "Data out"=w342:T3[], "CIFTag out"=w345:refnum<class "CIF_NIChn_Fifo_Power.lvclass">)  [unwired: 4 in, 2 out]
              }
              frame #2 {
                n94 = call <vilib>:"High Resolution Relative Seconds.vi"() -> ("relative seconds"=w348:dbl)
              }
            }
            n95 = Subtract(x=w323, y=w322) -> (x-y=w321:dbl)
            n96 = case shown="0" w316 {
              tunnel: w321 -> [_ w336]
              tunnel: w320 -> [w333 w335]
              tunnel: [w333 w334] -> w319
              frame 0 {
              }
              frame 1, Default {
                (unwired) u32 1 ("milliseconds to wait")
                n97 = Max & Min(x=w336, y=w335) -> (max(x,y)=w334:dbl)  [unwired: 1 out]
              }
            }
          }
        }
        "max TO" <- w292
        n98 = node-c288(w303) -> ()  [unwired: 1 out]
        n99 = node-c288(w301) -> ()  [unwired: 1 out]
        n100 = Subtract(x=w300, y=w299) -> (x-y=w298:dbl)
        n101 = call-dynamic "Destroy.vi"("error in (no error)"=w277, "CIFTag in"=w278) -> ("error out"=w276:errorcluster)  [unwired: 8 in, 1 out]
        n102 = Divide(x=w298, y=w297) -> (x/y=w294:dbl)
        "avg TO" <- w294
        n103 = call-dynamic "Destroy.vi"("error in (no error)"=w276, "CIFTag in"=w275) -> ("error out"=w274:errorcluster)  [unwired: 8 in, 1 out]
        n104 = Less?(x=w292, y=3e-05) -> (x < y?=w290:bool)
        n105 = Less?(x=w294, y=5e-07) -> ()  [unwired: 1 out]
      }
      frame 3 {
        n106 = call <vilib>:"Create NI GUID.vi"() -> ("NI GUID"=w406:string)
        n107 = call <vilib>:"Create NI GUID.vi"() -> ("NI GUID"=w411:string)
        n108 = call-dynamic "Create.vi"("Direction"=w410, "error in (no error)"=w412, "Custom Config Data"=w404, "Name"=w406, "CIFTag in"=w408) -> ("error out"=w413:errorcluster, "CIFTag out"=w399:refnum<class "CIF_NIChn_Fifo_Power.lvclass">)  [unwired: 5 in]
        n109 = call-dynamic "Create.vi"("Direction"=w409, "error in (no error)"=w413, "Custom Config Data"=w404, "Name"=w411, "CIFTag in"=w408) -> ("error out"=w405:errorcluster, "CIFTag out"=w407:refnum<class "CIF_NIChn_Fifo_Power.lvclass">)  [unwired: 5 in]
        n110 = call-dynamic "Connect.vi"("error in (no error)"=w405, "Connection Name"=w406, "CIFTag in"=w407) -> ("error out"=w397:errorcluster, "CIFTag out"=w403:refnum<class "CIF_NIChn_Fifo_Power.lvclass">)  [unwired: 7 in]
        n111 = flat-sequence {
          tunnel: w397 -> [w430]
          tunnel: [w430] -> w396
          frame #0 {
            n112 = Wait (ms)(milliseconds to wait=u32 100) -> ()  [unwired: 1 out]
          }
        }
        n113 = node-c288() -> (w428:T4)
        n114 = node-c288() -> (w426:T4)
        n115 = timed-loop {
          timing: w428 -> [_]
          timing-out: [_] -> w427
          tunnel: w403 -> [w497]
          tunnel: w396 -> [w496]
          tunnel: [w492] -> w420
          tunnel: [w490] -> w419
          tunnel: [w488] -> w424
          tunnel: [w487] -> w423
          tunnel: [w486] -> w421
          tunnel: [w484] -> w395
          stop <- TRUE stop-if-true
          n116 = flat-sequence {
            tunnel: w496 -> [w499]
            tunnel: w497 -> [w500]
            tunnel: [w500] -> w494
            tunnel: [w499] -> w493
            tunnel: [w498] -> w487
            tunnel: w494 -> [w506]
            tunnel: w493 -> [w505]
            tunnel: [w504] -> w491
            tunnel: [w503] -> w489
            tunnel: [w502] -> w485
            tunnel: [w501] -> w483
            tunnel: [w517] -> w492
            tunnel: w491 -> [w517]
            tunnel: [w516] -> w490
            tunnel: w489 -> [w516]
            tunnel: [w515] -> w488
            tunnel: [w514] -> w486
            tunnel: w485 -> [w514]
            tunnel: [w513] -> w484
            tunnel: w483 -> [w513]
            frame #0 {
              n117 = call <vilib>:"High Resolution Relative Seconds.vi"() -> ("relative seconds"=w498:dbl)
            }
            frame #1 {
              w502 = 1000
              n118 = for {
                N: w502 -> [_]
                shift-right: [w511] -> w504
                shift-left: w506 -> [w512]
                shift-right: [w509] -> w503
                shift-left: w505 -> [w510]
                shift-right: [w508] -> _
                shift-left: _ -> [_]
                tunnel: [w507] -> w501
                n119 = call-dynamic "Read Power FIFO.vi"("error in (no error)"=w510, "CIFTag in"=w512) -> ("error out"=w509:errorcluster, "timed out?"=w507:bool, "Data out"=w508:T3[], "CIFTag out"=w511:refnum<class "CIF_NIChn_Fifo_Power.lvclass">)  [unwired: 5 in, 1 out]
              }
            }
            frame #2 {
              n120 = call <vilib>:"High Resolution Relative Seconds.vi"() -> ("relative seconds"=w515:dbl)
            }
          }
        }
        "timed out? 4" <- w395
        n121 = timed-loop {
          timing: w426 -> [_]
          timing-out: [_] -> w425
          tunnel: w420 -> [w443]
          tunnel: w419 -> [w442]
          tunnel: [w440] -> w402
          tunnel: [w439] -> w401
          tunnel: [w436] -> w416
          stop <- TRUE stop-if-true
          n122 = for {
            N: 1000 -> [_]
            shift-right: [w455] -> w440
            shift-left: w443 -> [w457]
            shift-right: [w454] -> w439
            shift-left: w442 -> [w456]
            shift-right: [w448] -> w436
            shift-left: 0.0 -> [w449]
            shift-right: [w447] -> _
            shift-left: _ -> [w453]
            i -> [w445]
            n123 = flat-sequence {
              tunnel: w456 -> [w468]
              tunnel: w457 -> [w469]
              tunnel: [w469] -> w461
              tunnel: [w468] -> w460
              tunnel: [w467] -> w451
              tunnel: w453 -> [w466]
              tunnel: [w466] -> w459
              tunnel: w461 -> [w474]
              tunnel: w460 -> [w472]
              tunnel: [w473] -> w458
              tunnel: w459 -> [_]
              tunnel: [w470] -> w446
              tunnel: [w471] -> w444
              tunnel: [w478] -> w455
              tunnel: w458 -> [w478]
              tunnel: [w477] -> w454
              tunnel: [w476] -> w452
              tunnel: [w475] -> w447
              tunnel: w446 -> [w475]
              tunnel: w444 -> [w477]
              frame #0 {
                n124 = call <vilib>:"High Resolution Relative Seconds.vi"() -> ("relative seconds"=w467:dbl)
              }
              frame #1 {
                n125 = call-dynamic "Read Power FIFO.vi"("error in (no error)"=w472, "CIFTag in"=w474) -> ("error out"=w471:errorcluster, "Data out"=w470:T3[], "CIFTag out"=w473:refnum<class "CIF_NIChn_Fifo_Power.lvclass">)  [unwired: 5 in, 2 out]
              }
              frame #2 {
                n126 = call <vilib>:"High Resolution Relative Seconds.vi"() -> ("relative seconds"=w476:dbl)
              }
            }
            n127 = Subtract(x=w452, y=w451) -> (x-y=w450:dbl)
            n128 = case shown="0" w445 {
              tunnel: w450 -> [_ w465]
              tunnel: w449 -> [w462 w464]
              tunnel: [w462 w463] -> w448
              frame 0 {
              }
              frame 1, Default {
                (unwired) u32 1 ("milliseconds to wait")
                n129 = Max & Min(x=w465, y=w464) -> (max(x,y)=w463:dbl)  [unwired: 1 out]
              }
            }
          }
        }
        "max big channel" <- w416
        n130 = while {
          tunnel: w399 -> [w434]
          i -> [w435]
          stop <- w433 stop-if-true
          n131 = To Double Precision Float(number=w435) -> ()  [unwired: 1 out]
          n132 = call-dynamic "Write Power FIFO.vi"("Data In"=T3[] [{"measurement"=array[100001 elements], "dT"=0.0, "Timestamp"=0}, {"measurement"=array[100001 elements], "dT"=5.2, "Timestamp"=523}], "CIFTag in"=w434) -> ("error out"=w433:errorcluster)  [unwired: 6 in, 3 out]
          n133 = Wait (ms)(milliseconds to wait=u32 1) -> ()  [unwired: 1 out]
        }
        n134 = node-c288(w427) -> ()  [unwired: 1 out]
        n135 = node-c288(w425) -> ()  [unwired: 1 out]
        n136 = Subtract(x=w424, y=w423) -> (x-y=w422:dbl)
        n137 = call-dynamic "Destroy.vi"("error in (no error)"=w401, "CIFTag in"=w402) -> ("error out"=w400:errorcluster)  [unwired: 8 in, 1 out]
        n138 = Divide(x=w422, y=w421) -> (x/y=w418:dbl)
        "avg big channel" <- w418
        n139 = call-dynamic "Destroy.vi"("error in (no error)"=w400, "CIFTag in"=w399) -> ("error out"=w398:errorcluster)  [unwired: 8 in, 1 out]
        n140 = Less?(x=w416, y=0.002) -> (x < y?=w414:bool)
        n141 = Less?(x=w418, y=5e-07) -> ()  [unwired: 1 out]
      }
    }
  }
  "error out" <- w10
  n142 = And Array Elements(Boolean array=w8) -> (logical AND=→"pass":bool)
